vi "PDF errors.vi"(5 "code":i32, 7 "Additionnal information":string, 11 "error in (no error)":errorcluster) -> (15 "error out":errorcluster)   [LabVIEW 2012]
doc: "Version 1.0\nDeveloped by Jean-Marc Simard\nCopyright © 2010, Exaprom Inc.\nAll rights reserved.\nLicense: BSD\n\nWith iTextSharp 4.1.6 (http://itextsharp.sourceforge.net)\nunder Mozilla Public License Version 1.1\n(http://www.mozilla.org/MPL/MPL-1.1.html)"
panel:
  in  "Call Chain (T)?":bool=TRUE
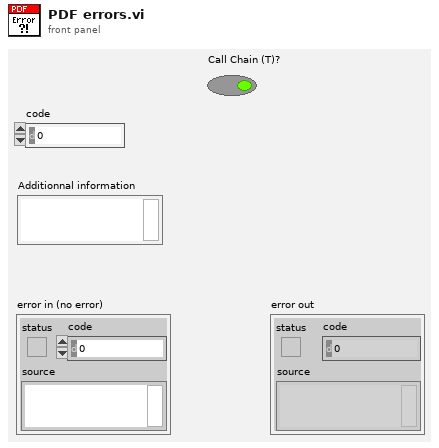
[diagram p1: front panel]
types:
  T1 = cluster{"status":bool, "index of element":i32, string}
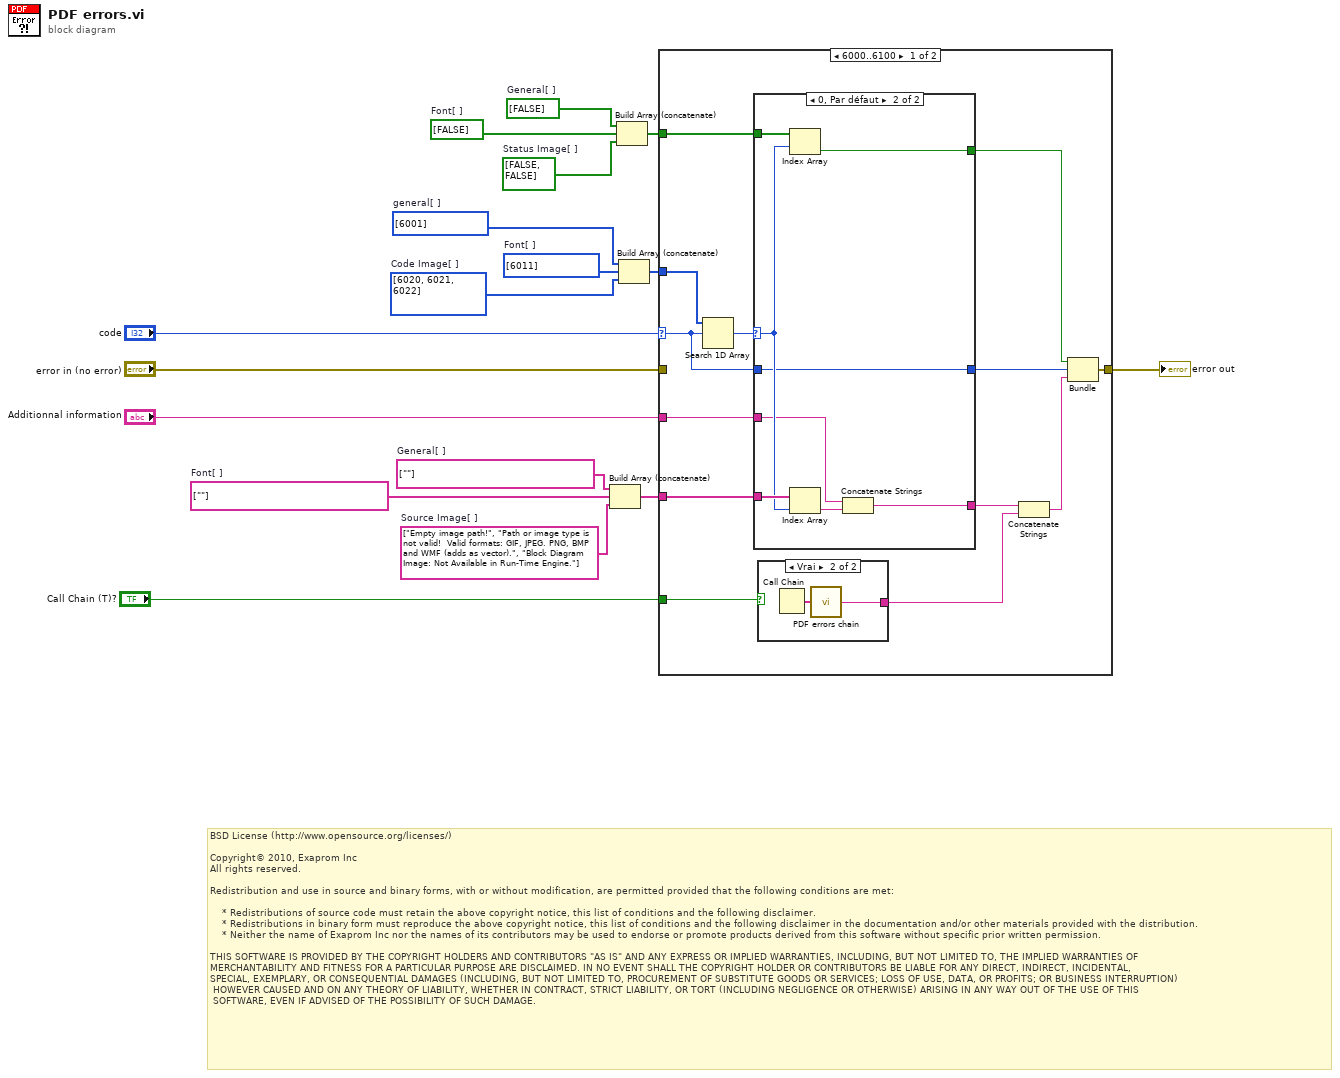
[diagram p0: block diagram]
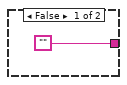
[diagram p2: hidden frame]
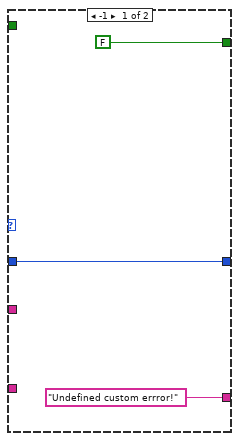
[diagram p3: hidden frame]
diagram:
  w7 = string[] [""]  # Font[ ]
  w6 = i32[] [6011]  # Font[ ]
  w3 = bool[] [FALSE]  # Font[ ]
  w10 = string[] [""]  # General[ ]
  w9 = i32[] [6001]  # general[ ]
  w8 = bool[] [FALSE]  # General[ ]
  w2 = bool[] [FALSE, FALSE]  # Status Image[ ]
  w4 = string[] ["Empty image path!", "Path or image type is not valid!  Valid formats: GIF, JPEG. PNG, BMP and WMF (adds as vector).", "Block Diagram Image: Not Available in Run-Time Engine."]  # Source Image[ ]
  w5 = i32[] [6020, 6021, 6022]  # Code Image[ ]
  # "BSD License (http://www.opensource.org/licenses/)\n\nCopyright© 2010, Exaprom Inc\nAll rights reserved.\n\nRedistribution and use in source and binary forms, with or without modification, are permitted provided that the following conditions are met:\n\n    * Redistributions of source code must retain the above copyright notice, this list of conditions and the following disclaimer.\n    * Redistributions in binary form must reproduce the above copyright notice, this list of conditions and the following disclaimer in the documentation and/or other materials provided with the distribution.\n    * Neither the name of Exaprom Inc nor the names of its contributors may be used to endorse or promote products derived from this software without specific prior written permission.\n\nTHIS SOFTWARE IS PROVIDED BY THE COPYRIGHT HOLDERS AND CONTRIBUTORS \"AS IS\" AND ANY EXPRESS OR IMPLIED WARRANTIES, INCLUDING, BUT NOT LIMITED TO, THE IMPLIED WARRANTIES OF \nMERCHANTABILITY AND FITNESS FOR A PARTICULAR PURPOSE ARE DISCLAIMED. IN NO EVENT SHALL THE COPYRIGHT HOLDER OR CONTRIBUTORS BE LIABLE FOR ANY DIRECT, INDIRECT, INCIDENTAL,\nSPECIAL, EXEMPLARY, OR CONSEQUENTIAL DAMAGES (INCLUDING, BUT NOT LIMITED TO, PROCUREMENT OF SUBSTITUTE GOODS OR SERVICES; LOSS OF USE, DATA, OR PROFITS; OR BUSINESS INTERRUPTION)\n HOWEVER CAUSED AND ON ANY THEORY OF LIABILITY, WHETHER IN CONTRACT, STRICT LIABILITY, OR TORT (INCLUDING NEGLIGENCE OR OTHERWISE) ARISING IN ANY WAY OUT OF THE USE OF THIS\n SOFTWARE, EVEN IF ADVISED OF THE POSSIBILITY OF SUCH DAMAGE."
  n1 = Build Array (concatenate)(w10, w7, w4) -> (w11:string[])
  n2 = Build Array (concatenate)(w8, w3, w2) -> (w13:bool[])
  n3 = Build Array (concatenate)(w9, w6, w5) -> (w12:i32[])
  n4 = case shown="6000..6100" "code" {
    selector: "code" -> [w26 _]
    tunnel: w13 -> [w27 _]
    tunnel: w11 -> [w28 _]
    tunnel: w12 -> [w30 _]
    tunnel: "error in (no error)" -> [_ w45]
    tunnel: [w22 w45] -> w15
    tunnel: "Additionnal information" -> [w21 _]
    tunnel: "Call Chain (T)?" -> [w20 _]
    frame 6000..6100 {
      n5 = Search 1D Array(1D array=w30, element=w26) -> (index of element=w29:i32)  [unwired: 1 out]
      n6 = case shown="0, Par défaut" w29 {
        selector: w29 -> [_ w42]
        tunnel: w28 -> [_ w44]
        tunnel: w27 -> [_ w43]
        tunnel: w26 -> [w36 w41]
        tunnel: [w36 w41] -> w25
        tunnel: [FALSE ("status") w40] -> w24
        tunnel: ["Undefined custom errror!" ("source") w38] -> w23
        tunnel: w21 -> [_ w37]
        frame -1 {
        }
        frame 0, Default {
          n7 = Index Array(array=w43, index=w42) -> (element=w40:bool)
          n8 = Index Array(array=w44, index=w42) -> (element=w39:string)
          n9 = Concatenate Strings(w37, w39) -> (w38:string)
        }
      }
      n10 = case shown="Vrai" w20 {
        tunnel: ["" w32] -> w18
        frame False {
        }
        frame True {
          n11 = Call Chain() -> (call chain=w33:string[])
          n12 = call "PDF errors chain.vi"("call chain"=w33) -> ("String chain"=w32:string)  [unwired: 14 out]
        }
      }
      n13 = Concatenate Strings(w23, w18) -> (w19:string)
      n14 = Bundle("status"=w24, "index of element"=w25, w19) -> (w22:T1)  [unwired: 1 out]
    }
    frame 0, Default {
    }
  }
  "error out" <- w15
